vi "fromdB.vi"(1 "Input (dB (10))":dbl) -> (0 "Output":dbl)   [LabVIEW 2009]
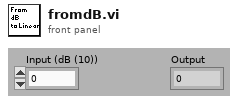
[diagram p1: front panel]
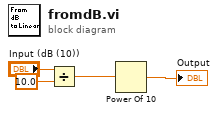
[diagram p0: block diagram]
diagram:
  n1 = Divide(x="Input (dB (10))", y=10.0) -> (x/y=w2:dbl)
  n2 = Power Of 10(x=w2) -> (10^x=→"Output":dbl)
